vi "ValidateNumInSquare.vi"(8 "Number":i32, 9 "Column":i32, 10 "Row":i32, 11 "Board":i32[][](array[numeric])) -> (0 "Number":i32, 1 "Column":i32, 2 "Row":i32, 3 "Board":i32[][](array[numeric]), 4 "Valid in Square":bool)   [LabVIEW 2023]
doc: "Checks if Number is valid in the current Square\n\nInputs\n- Board: Current Board Configuration\n- Row: Row of current Cell\n- Column: Column of current Cell\n- Number: Number to try out in current Cell\n\nOutputs\n- Board: Current Board Configuration\n- Row: Row of current Cell\n- Column: Column of current Cell\n- Number: Number to try out in current Cell\n- Valid in Square: TRUE if Number is valid in current Square"
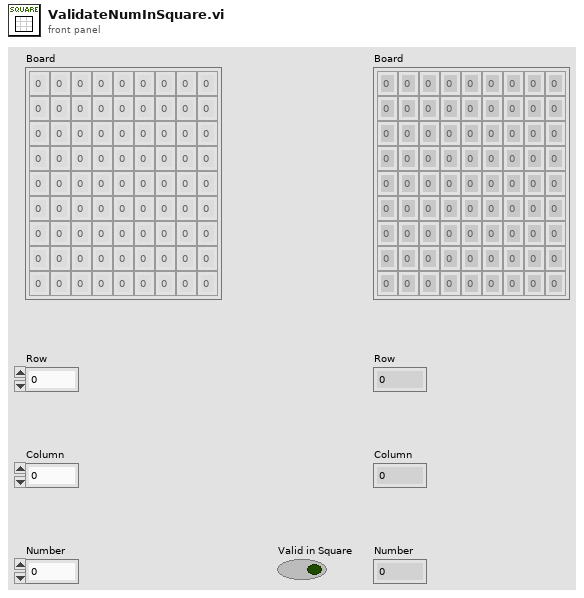
[diagram p1: front panel]
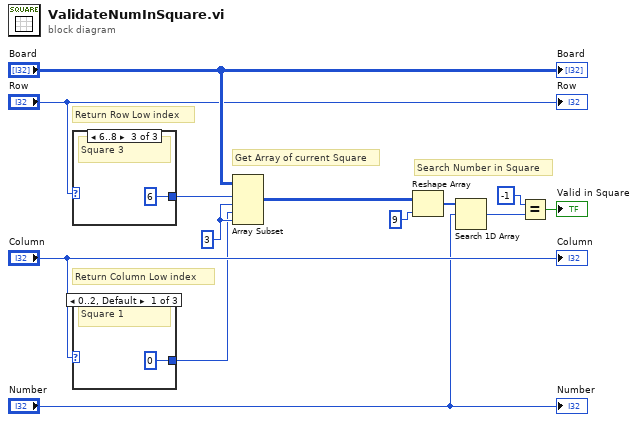
[diagram p0: block diagram]
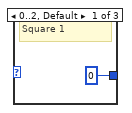
[diagram p2: hidden frame]
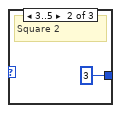
[diagram p3: hidden frame]
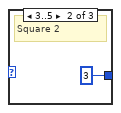
[diagram p4: hidden frame]
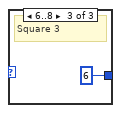
[diagram p5: hidden frame]
diagram:
  w8 = 3 ("length")
  # "Return Column Low index"
  # "Return Row Low index"
  # "Get Array of current Square"
  # "Search Number in Square"
  n1 = case shown="6..8" "Row" {
    tunnel: [0 ("Row") 3 ("Row") 6 ("Row")] -> w2
    frame 0..2, Default {
      # "Square 1"
    }
    frame 3..5 {
      # "Square 2"
    }
    frame 6..8 {
      # "Square 3"
    }
  }
  n2 = case shown="0..2, Default" "Column" {
    tunnel: [0 ("Row") 3 ("Row") 6 ("Row")] -> w3
    frame 0..2, Default {
      # "Square 1"
    }
    frame 3..5 {
      # "Square 2"
    }
    frame 6..8 {
      # "Square 3"
    }
  }
  n3 = Array Subset(array="Board", index (row)=w2, length (row)=w8, index (col)=w3, length (col)=w8) -> (w4:i32[][])
  n4 = Reshape Array(w4, 9 ("dimension size")) -> (w5:i32[])
  n5 = Search 1D Array(1D array=w5, element="Number") -> (index of element=w6:i32)  [unwired: 1 in]
  n6 = Equal?(x=-1, y=w6) -> (x = y?=→"Valid in Square":bool)
  "Board" <- "Board"
  "Column" <- "Column"
  "Number" <- "Number"
  "Row" <- "Row"
